vi "HEWH Extract Calibration Information.vi"(8 "error in (no error)":errorcluster, 11 "Top Header Data":string[][](array[string])) -> (0 "error out":errorcluster, 3 "Calibration Information":string[][](array[string]))   [LabVIEW 2023]
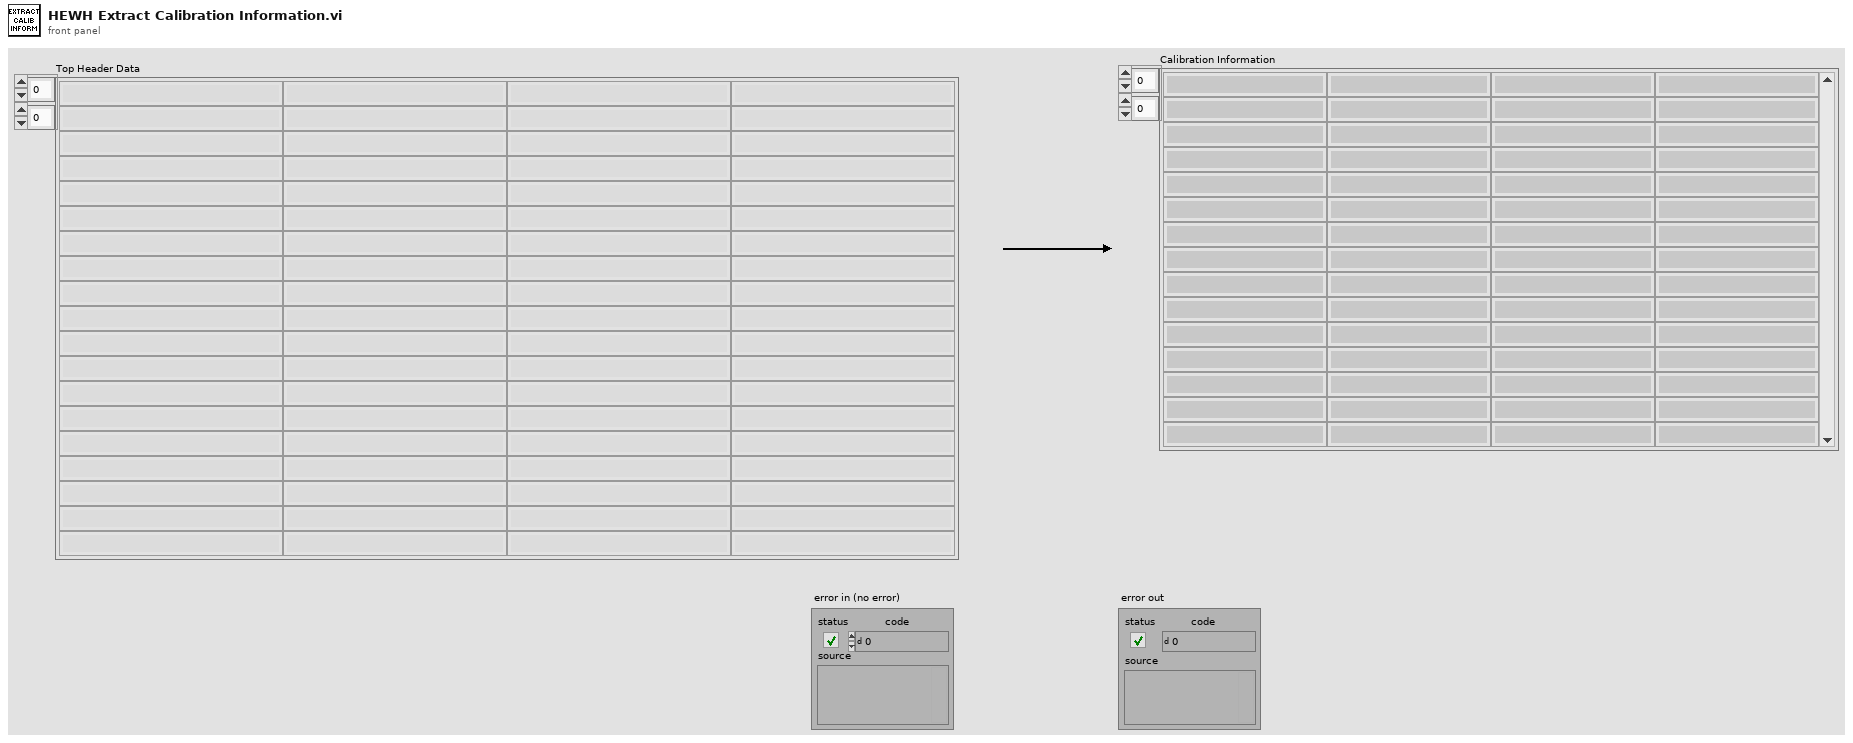
[diagram p1: front panel]
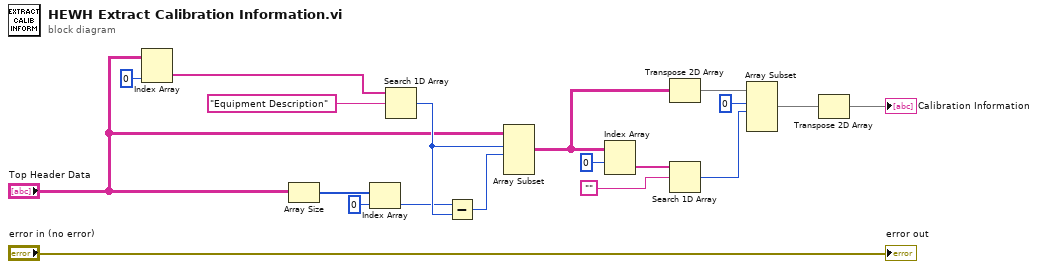
[diagram p0: block diagram]
diagram:
  n1 = Index Array(array="Top Header Data", index (col)=0 ("disabled index (col)")) -> (element=w2:string[])  [unwired: 1 in]
  n2 = Array Size(array="Top Header Data") -> (size(s)=w6:i32[])
  n3 = Index Array(array=w6, index=0) -> (element=w8:i32)
  n4 = Search 1D Array(1D array=w2, element="Equipment Description") -> (index of element=w9:i32)  [unwired: 1 in]
  n5 = Subtract(x=w8, y=w9) -> (x-y=w10:i32)
  n6 = Array Subset(array="Top Header Data", index (row)=w9, length (row)=w10) -> (w14:string[][])  [unwired: 2 in]
  n7 = Index Array(array=w14, index (row)=0) -> (element=w12:string[])  [unwired: 1 in]
  n8 = Transpose 2D Array(2D array=w14) -> (transposed array=w15:string[][])
  n9 = Search 1D Array(1D array=w12, element="") -> (index of element=w17:i32)  [unwired: 1 in]
  n10 = Array Subset(array=w15, index (row)=0 ("index"), length (row)=w17) -> (w18:string[][])  [unwired: 2 in]
  n11 = Transpose 2D Array(2D array=w18) -> (transposed array=→"Calibration Information":string[][])
  "error out" <- "error in (no error)"
